vi "IV_Sensor_Check.vi"(10 "Data":dbl[][](array[numeric])=[[1.0, -1.0, 15.0, -15.0], [2.0, -2.0, 30.0, -30.0], [3.0, -3.0, 45.0, -45.0], [4.0, -4.0, 60.0, -60.0]], 11 "Titles":string[](array[string])=["Bias", "Total", "Active", "Guard"]) -> (2 "Boolean Pass/Fail Array":bool[](array[boolean]), 3 "Test Check Names":string[](array[string]))   [LabVIEW 2009]
panel:
  out "Pass/Fail":T1
  out "Passed/Failed Tests":string[](array[string])
  out "Pass":bool
  out "Voltage Breakdown":bool
  out "avg-y 2":dbl
  out "Loop Iteration":i32
  out "avg-y":dbl
  out "avg-x":dbl
  out "Leakage Current Guardring":bool caption="Leakage Current Check Guard"
  out "Leakage Current Check Active":bool
  out "Leakage Current Check Total":bool
  out "150V Bias Check":bool
  out "element 5":dbl
  out "element 4":string
  out "Guadring":dbl[](array[numeric])
  out "element 3":string
  out "Active":dbl[](array[numeric])
  out "element 2":string
  out "Total":dbl[](array[numeric])
  out "element":string
  out "Bias":dbl[](array[numeric])
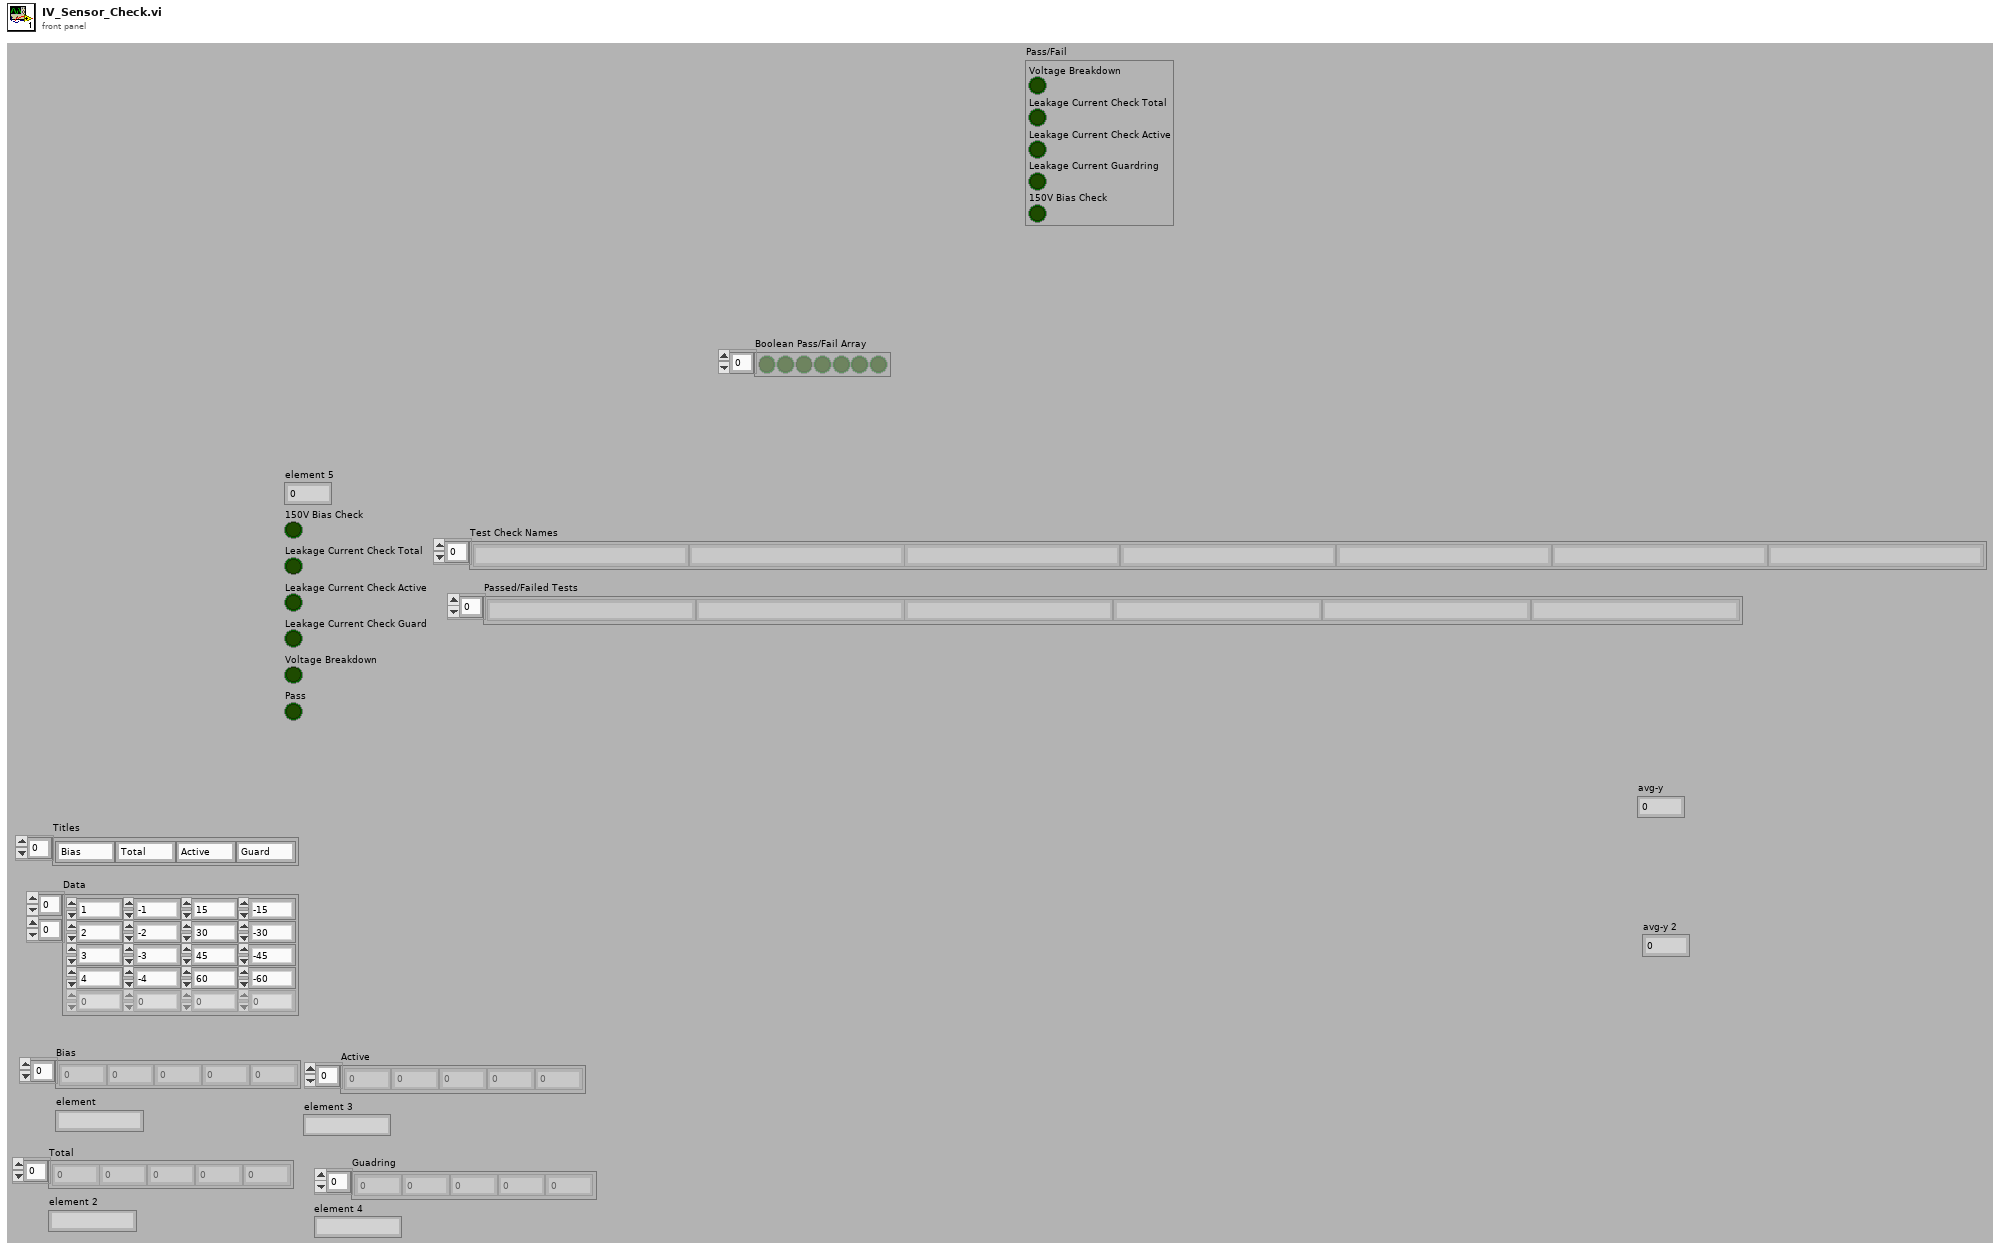
[diagram p1: front panel]
types:
  T1 = cluster{"Voltage Breakdown":bool, "Leakage Current Check Total":bool, "Leakage Current Check Active":bool, "Leakage Current Guardring":bool, "150V Bias Check":bool}
  T2 = cluster{"Numeric":dbl, "Numeric":dbl, "Numeric":dbl, "Numeric":dbl, "Numeric":dbl}
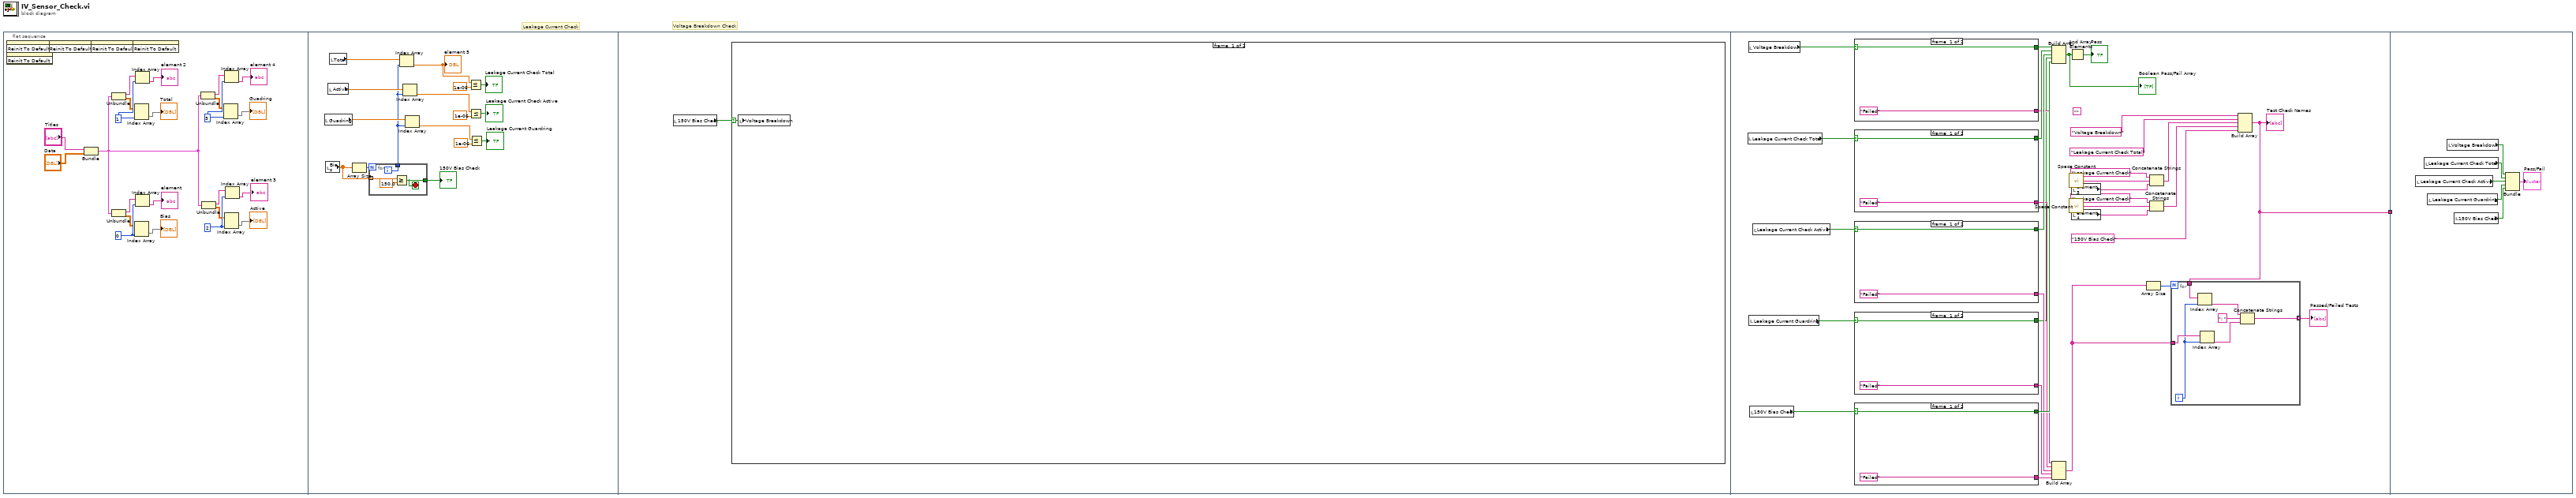
[diagram p0: block diagram]
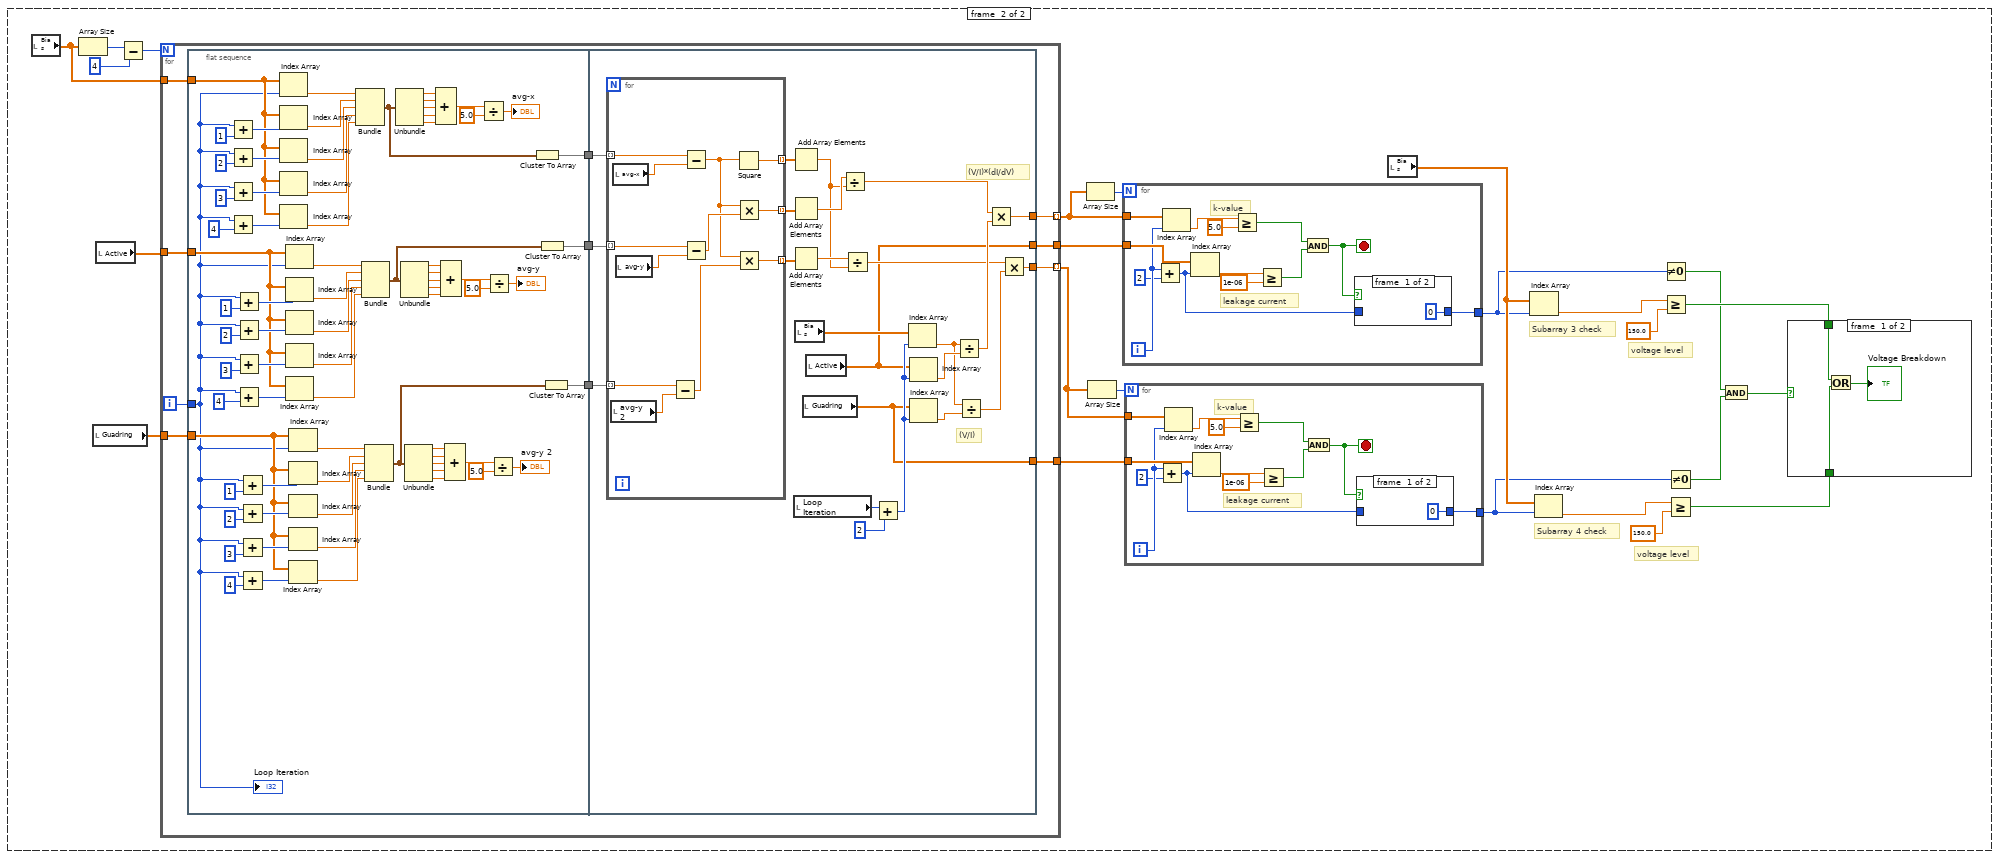
[diagram p2: hidden frame]
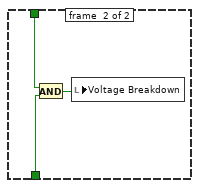
[diagram p3: hidden frame]
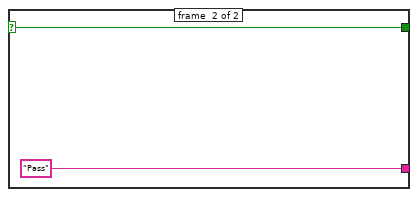
[diagram p6: hidden frame]
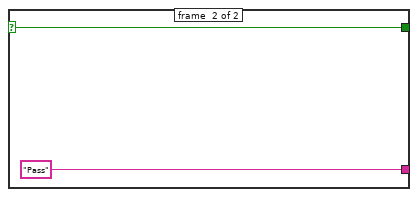
[diagram p7: hidden frame]
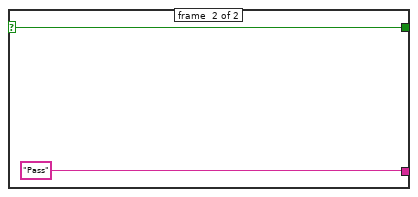
[diagram p8: hidden frame]
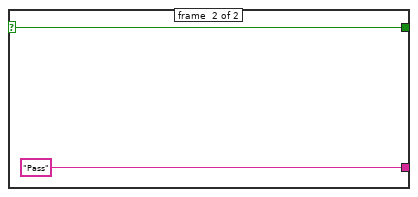
[diagram p9: hidden frame]
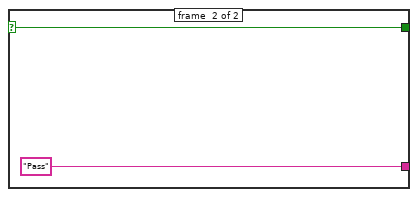
[diagram p10: hidden frame]
diagram:
  # "Voltage Breakdown Check"
  # "Leakage Current Check"
  n1 = flat-sequence {
    tunnel: [w228] -> w1
    tunnel: w1 -> [_]
    frame #0 {
      w23 = u32 3 ("milliseconds to wait")
      w18 = u32 2 ("milliseconds to wait")
      w13 = u32 1 ("milliseconds to wait")
      w8 = u32 0 ("milliseconds to wait")
      n2 = invoke on="Leakage Current Check Total" class="Bool (strict)" method="Reinit To Default"() -> ()  [unwired: 3 in, 3 out]
      n3 = invoke on="Voltage Breakdown" class="Bool (strict)" method="Reinit To Default"() -> ()  [unwired: 3 in, 3 out]
      n4 = invoke on="Leakage Current Check Active" class="Bool (strict)" method="Reinit To Default"() -> ()  [unwired: 3 in, 3 out]
      n5 = Bundle("Titles"="Titles", "Data"="Data") -> (w24:cluster{"Titles":string[], "Data":dbl[][]})  [unwired: 1 in]
      n6 = invoke on="Leakage Current Guardring" class="Bool (strict)" method="Reinit To Default"() -> ()  [unwired: 3 in, 3 out]
      n7 = Unbundle(w24) -> ("Titles"=w11:string[], "Data"=w12:dbl[][])
      n8 = Unbundle(w24) -> ("Titles"=w6:string[], "Data"=w7:dbl[][])
      n9 = invoke on="150V Bias Check" class="Bool (strict)" method="Reinit To Default"() -> ()  [unwired: 3 in, 3 out]
      n10 = Index Array(array=w12, index (col)=w13) -> (element=→"Total":dbl[])  [unwired: 1 in]
      n11 = Index Array(array=w7, index (col)=w8) -> (element=→"Bias":dbl[])  [unwired: 1 in]
      n12 = Index Array(array=w11, index=w13) -> (element=→"element 2":string)
      n13 = Index Array(array=w6, index=w8) -> (element=→"element":string)
      n14 = Unbundle(w24) -> ("Titles"=w21:string[], "Data"=w22:dbl[][])
      n15 = Unbundle(w24) -> ("Titles"=w16:string[], "Data"=w17:dbl[][])
      n16 = Index Array(array=w22, index (col)=w23) -> (element=→"Guadring":dbl[])  [unwired: 1 in]
      n17 = Index Array(array=w17, index (col)=w18) -> (element=→"Active":dbl[])  [unwired: 1 in]
      n18 = Index Array(array=w21, index=w23) -> (element=→"element 4":string)
      n19 = Index Array(array=w16, index=w18) -> (element=→"element 3":string)
    }
    frame #1 {
      n20 = local read "Guadring"() -> (w29:dbl[])
      n21 = local read "Bias"() -> (w39:dbl[])
      n22 = local read "Active"() -> (w33:dbl[])
      n23 = local read "Total"() -> (w34:dbl[])
      n24 = Array Size(array=w39) -> (size(s)=w40:i32)
      n25 = for {
        N: w40 -> [_]
        tunnel: w39 -> [w43] mode=indexing
        tunnel: [w42] -> w28
        tunnel: [w41] -> w38
        i -> [w42]
        stop <- w41 stop-if-true
        n26 = Greater Or Equal?(x=w43, y=150.0 ("element")) -> (x >= y?=w41:bool)
      }
      "150V Bias Check" <- w38
      n27 = Index Array(array=w34, index=w28) -> (element=w37:dbl)
      "element 5" <- w37
      n28 = Index Array(array=w33, index=w28) -> (element=w30:dbl)
      n29 = Index Array(array=w29, index=w28) -> (element=w25:dbl)
      n30 = Less Or Equal?(x=w37, y=1e-06) -> (x <= y?=→"Leakage Current Check Total":bool)
      n31 = Less Or Equal?(x=w30, y=1e-06) -> (x <= y?=→"Leakage Current Check Active":bool)
      n32 = Less Or Equal?(x=w25, y=1e-06) -> (x <= y?=→"Leakage Current Guardring":bool)
    }
    frame #2 {
      n33 = local read "150V Bias Check"() -> (w45:bool)
      n34 = case shown="True" w45 {
        selector: w45 -> [w46 _]
        frame #0 {
          n35 = local write "Voltage Breakdown"(w46) -> ()
        }
        frame #1 {
          # "voltage level"
          # "voltage level"
          # "Subarray 4 check"
          # "Subarray 3 check"
          n36 = local read "Bias"() -> (w67:dbl[])
          n37 = Array Size(array=w67) -> (size(s)=w69:i32)
          n38 = local read "Guadring"() -> (w65:dbl[])
          n39 = local read "Active"() -> (w66:dbl[])
          n40 = Subtract(x=w69, y=4) -> (x-y=w70:i32)
          n41 = for {
            N: w70 -> [_]
            tunnel: w67 -> [w117]
            tunnel: w66 -> [w116]
            tunnel: w65 -> [w112]
            tunnel: [w110] -> w62 mode=indexing
            tunnel: [w109] -> w58 mode=indexing
            tunnel: [w108] -> w64
            tunnel: [w107] -> w60
            i -> [w113]
            n42 = flat-sequence {
              tunnel: w113 -> [w122]
              tunnel: w117 -> [w180]
              tunnel: w116 -> [w150]
              tunnel: [w148] -> w115
              tunnel: [w146] -> w114
              tunnel: w112 -> [w124]
              tunnel: [w123] -> w111
              tunnel: w115 -> [w214]
              tunnel: w114 -> [w213]
              tunnel: w111 -> [w203]
              tunnel: [w194] -> w110
              tunnel: [w193] -> w109
              tunnel: [w192] -> w108
              tunnel: [w191] -> w107
              frame #0 {
                n43 = Add(x=w122, y=1) -> (x+y=w188:i32)
                n44 = Add(x=w122, y=2) -> (x+y=w189:i32)
                n45 = Add(x=w122, y=3) -> (x+y=w190:i32)
                n46 = Add(x=w122, y=4) -> (x+y=w119:i32)
                n47 = Add(x=w122, y=1) -> (x+y=w167:i32)
                n48 = Add(x=w122, y=2) -> (x+y=w168:i32)
                n49 = Add(x=w122, y=3) -> (x+y=w169:i32)
                n50 = Add(x=w122, y=4) -> (x+y=w120:i32)
                n51 = Add(x=w122, y=1) -> (x+y=w143:i32)
                n52 = Add(x=w122, y=2) -> (x+y=w144:i32)
                n53 = Add(x=w122, y=3) -> (x+y=w145:i32)
                n54 = Add(x=w122, y=4) -> (x+y=w121:i32)
                n55 = Index Array(array=w180, index=w122) -> (element=w183:dbl)
                n56 = Index Array(array=w180, index=w188) -> (element=w178:dbl)
                n57 = Index Array(array=w180, index=w189) -> (element=w179:dbl)
                n58 = Index Array(array=w180, index=w190) -> (element=w181:dbl)
                n59 = Index Array(array=w180, index=w119) -> (element=w182:dbl)
                n60 = Index Array(array=w150, index=w122) -> (element=w163:dbl)
                n61 = Index Array(array=w150, index=w167) -> (element=w159:dbl)
                n62 = Index Array(array=w150, index=w168) -> (element=w160:dbl)
                n63 = Index Array(array=w150, index=w169) -> (element=w161:dbl)
                n64 = Index Array(array=w150, index=w120) -> (element=w162:dbl)
                n65 = Index Array(array=w124, index=w122) -> (element=w138:dbl)
                n66 = Index Array(array=w124, index=w143) -> (element=w134:dbl)
                n67 = Index Array(array=w124, index=w144) -> (element=w135:dbl)
                n68 = Index Array(array=w124, index=w145) -> (element=w136:dbl)
                n69 = Index Array(array=w124, index=w121) -> (element=w137:dbl)
                n70 = Bundle("Numeric"=w183, "Numeric"=w178, "Numeric"=w179, "Numeric"=w181, "Numeric"=w182) -> (w149:T2)  [unwired: 1 in]
                n71 = Bundle("Numeric"=w163, "Numeric"=w159, "Numeric"=w160, "Numeric"=w161, "Numeric"=w162) -> (w147:T2)  [unwired: 1 in]
                n72 = Bundle("Numeric"=w138, "Numeric"=w134, "Numeric"=w135, "Numeric"=w136, "Numeric"=w137) -> (w125:T2)  [unwired: 1 in]
                n73 = Unbundle(w149) -> ("Numeric"=w171:dbl, "Numeric"=w172:dbl, "Numeric"=w173:dbl, "Numeric"=w174:dbl, "Numeric"=w175:dbl)
                n74 = Unbundle(w147) -> ("Numeric"=w152:dbl, "Numeric"=w153:dbl, "Numeric"=w154:dbl, "Numeric"=w155:dbl, "Numeric"=w156:dbl)
                n75 = Unbundle(w125) -> ("Numeric"=w127:dbl, "Numeric"=w128:dbl, "Numeric"=w129:dbl, "Numeric"=w130:dbl, "Numeric"=w131:dbl)
                n76 = Compound Arithmetic op=ADD(w171, w172, w173, w174, w175) -> (w170:dbl)
                n77 = Compound Arithmetic op=ADD(w152, w153, w154, w155, w156) -> (w151:dbl)
                n78 = Compound Arithmetic op=ADD(w127, w128, w129, w130, w131) -> (w126:dbl)
                n79 = Divide(x=w170, y=5.0) -> (x/y=→"avg-x":dbl)
                n80 = Divide(x=w151, y=5.0) -> (x/y=→"avg-y":dbl)
                n81 = Divide(x=w126, y=5.0) -> (x/y=→"avg-y 2":dbl)
                n82 = Cluster To Array(cluster=w149) -> (array=w148:dbl[])
                n83 = Cluster To Array(cluster=w147) -> (array=w146:dbl[])
                n84 = Cluster To Array(cluster=w125) -> (array=w123:dbl[])
                "Loop Iteration" <- w122
              }
              frame #1 {
                # "(V/I)*(dI/dV)"
                # "(V/I)"
                n85 = for {
                  tunnel: w214 -> [w226] mode=indexing
                  tunnel: w213 -> [w224] mode=indexing
                  tunnel: [w221] -> w212 mode=indexing
                  tunnel: [w220] -> w211 mode=indexing
                  tunnel: w203 -> [w219] mode=indexing
                  tunnel: [w215] -> w201 mode=indexing
                  n86 = local read "avg-y 2"() -> (w218:dbl)
                  n87 = local read "avg-x"() -> (w225:dbl)
                  n88 = local read "avg-y"() -> (w223:dbl)
                  n89 = Subtract(x=w219, y=w218) -> (x-y=w216:dbl)
                  n90 = Subtract(x=w226, y=w225) -> (x-y=w217:dbl)
                  n91 = Subtract(x=w224, y=w223) -> (x-y=w222:dbl)
                  n92 = Square(x=w217) -> (x^2=w221:dbl)
                  n93 = Multiply(x=w217, y=w222) -> (x*y=w220:dbl)
                  n94 = Multiply(x=w217, y=w216) -> (x*y=w215:dbl)
                }
                n95 = Add Array Elements(numeric array=w212) -> (sum=w199:dbl)
                n96 = Add Array Elements(numeric array=w211) -> (sum=w210:dbl)
                n97 = Add Array Elements(numeric array=w201) -> (sum=w200:dbl)
                n98 = local read "Loop Iteration"() -> (w209:i32)
                n99 = local read "Bias"() -> (w207:dbl[])
                n100 = local read "Guadring"() -> (w191:dbl[])
                n101 = local read "Active"() -> (w192:dbl[])
                n102 = Divide(x=w210, y=w199) -> (x/y=w205:dbl)
                n103 = Divide(x=w200, y=w199) -> (x/y=w196:dbl)
                n104 = Add(x=w209, y=2) -> (x+y=w202:i32)
                n105 = Index Array(array=w207, index=w202) -> (element=w197:dbl)
                n106 = Index Array(array=w192, index=w202) -> (element=w206:dbl)
                n107 = Index Array(array=w191, index=w202) -> (element=w198:dbl)
                n108 = Divide(x=w197, y=w206) -> (x/y=w204:dbl)
                n109 = Divide(x=w197, y=w198) -> (x/y=w195:dbl)
                n110 = Multiply(x=w205, y=w204) -> (x*y=w194:dbl)
                n111 = Multiply(x=w196, y=w195) -> (x*y=w193:dbl)
              }
            }
          }
          n112 = Array Size(array=w62) -> (size(s)=w63:i32)
          n113 = Array Size(array=w58) -> (size(s)=w59:i32)
          n114 = for {
            N: w63 -> [_]
            tunnel: w62 -> [w104]
            tunnel: w64 -> [w103]
            tunnel: [w93] -> w52
            i -> [w102]
            stop <- w92 stop-if-true
            # "leakage current"
            # "k-value"
            n115 = Add(x=w102, y=2) -> (x+y=w94:i32)
            n116 = Index Array(array=w104, index=w102) -> (element=w100:dbl)
            n117 = Index Array(array=w103, index=w94) -> (element=w99:dbl)
            n118 = Greater Or Equal?(x=w100, y=5.0) -> (x >= y?=w98:bool)
            n119 = Greater Or Equal?(x=w99, y=1e-06) -> (x >= y?=w97:bool)
            n120 = And(x=w98, y=w97) -> (x .and. y?=w92:bool)
            n121 = case shown="False" w92 {
              tunnel: w94 -> [_ w106]
              tunnel: [0 w106] -> w93
              frame #0 {
              }
              frame #1 {
              }
            }
          }
          n122 = for {
            N: w59 -> [_]
            tunnel: w58 -> [w89]
            tunnel: w60 -> [w88]
            tunnel: [w78] -> w53
            i -> [w87]
            stop <- w77 stop-if-true
            # "leakage current"
            # "k-value"
            n123 = Add(x=w87, y=2) -> (x+y=w79:i32)
            n124 = Index Array(array=w89, index=w87) -> (element=w85:dbl)
            n125 = Index Array(array=w88, index=w79) -> (element=w84:dbl)
            n126 = Greater Or Equal?(x=w85, y=5.0) -> (x >= y?=w83:bool)
            n127 = Greater Or Equal?(x=w84, y=1e-06) -> (x >= y?=w82:bool)
            n128 = And(x=w83, y=w82) -> (x .and. y?=w77:bool)
            n129 = case shown="False" w77 {
              tunnel: w79 -> [_ w91]
              tunnel: [0 w91] -> w78
              frame #0 {
              }
              frame #1 {
              }
            }
          }
          n130 = local read "Bias"() -> (w56:dbl[])
          n131 = Index Array(array=w56, index=w52) -> (element=w55:dbl)
          n132 = Index Array(array=w56, index=w53) -> (element=w54:dbl)
          n133 = Not Equal To 0?(x=w52) -> (x != 0?=w49:bool)
          n134 = Greater Or Equal?(x=w55, y=150.0) -> (x >= y?=w51:bool)
          n135 = Not Equal To 0?(x=w53) -> (x != 0?=w48:bool)
          n136 = Greater Or Equal?(x=w54, y=150.0) -> (x >= y?=w50:bool)
          n137 = And(x=w49, y=w48) -> (x .and. y?=w47:bool)
          n138 = case shown="False" w47 {
            tunnel: w51 -> [w72 w75]
            tunnel: w50 -> [w71 w74]
            frame #0 {
              n139 = Or(x=w72, y=w71) -> (x .or. y?=→"Voltage Breakdown":bool)
            }
            frame #1 {
              n140 = And(x=w75, y=w74) -> (x .and. y?=w76:bool)
              n141 = local write "Voltage Breakdown"(w76) -> ()
            }
          }
        }
      }
    }
    frame #3 {
      (unwired) ""
      n142 = local read "Leakage Current Check Total"() -> (w257:bool)
      n143 = local read "Voltage Breakdown"() -> (w258:bool)
      n144 = local read "Leakage Current Guardring"() -> (w255:bool)
      n145 = local read "150V Bias Check"() -> (w256:bool)
      n146 = local read "Leakage Current Check Active"() -> (w254:bool)
      n147 = case shown="False" w258 {
        selector: w258 -> [w283 w285]
        tunnel: [w283 w285] -> w253
        tunnel: ["Failed" "Pass"] -> w244
        frame #0 {
        }
        frame #1 {
        }
      }
      n148 = case shown="False" w257 {
        selector: w257 -> [w279 w281]
        tunnel: [w279 w281] -> w252
        tunnel: ["Failed" "Pass"] -> w245
        frame #0 {
        }
        frame #1 {
        }
      }
      n149 = case shown="False" w254 {
        selector: w254 -> [w267 w269]
        tunnel: [w267 w269] -> w251
        tunnel: ["Failed" "Pass"] -> w246
        frame #0 {
        }
        frame #1 {
        }
      }
      n150 = case shown="False" w255 {
        selector: w255 -> [w271 w273]
        tunnel: [w271 w273] -> w227
        tunnel: ["Failed" "Pass"] -> w247
        frame #0 {
        }
        frame #1 {
        }
      }
      n151 = case shown="False" w256 {
        selector: w256 -> [w275 w277]
        tunnel: [w275 w277] -> w250
        tunnel: ["Failed" "Pass"] -> w248
        frame #0 {
        }
        frame #1 {
        }
      }
      n152 = Build Array(w253, w252, w251, w227, w250) -> (w229:bool[])
      "Boolean Pass/Fail Array" <- w229
      n153 = Build Array(w244, w245, w246, w247, w248) -> (w231:string[])
      n154 = call <vilib>:"Space Constant.vi"() -> ("String"=w242:string)
      n155 = call <vilib>:"Space Constant.vi"() -> ("String"=w239:string)
      n156 = And Array Elements(Boolean array=w229) -> (logical AND=→"Pass":bool)
      n157 = local read "element 3"() -> (w241:string)
      n158 = local read "element 4"() -> (w238:string)
      n159 = Array Size(array=w231) -> (size(s)=w232:i32)
      n160 = Concatenate Strings("Leakage Current Check", w242, w241) -> (w235:string)
      n161 = Concatenate Strings("Leakage Current Check", w239, w238) -> (w234:string)
      n162 = Build Array("Voltage Breakdown", "Leakage Current Check Total", w235, w234, "150V Bias Check") -> (w228:string[])
      "Test Check Names" <- w228
      n163 = for {
        N: w232 -> [_]
        tunnel: w228 -> [w265]
        tunnel: w231 -> [w264]
        tunnel: [w260] -> w230 mode=indexing
        i -> [w259]
        n164 = Index Array(array=w265, index=w259) -> (element=w263:string)
        n165 = Index Array(array=w264, index=w259) -> (element=w262:string)
        n166 = Concatenate Strings(w263, ": " ("string"), w262) -> (w260:string)
      }
      "Passed/Failed Tests" <- w230
    }
    frame #4 {
      n167 = local read "Leakage Current Check Active"() -> (w289:bool)
      n168 = local read "Leakage Current Check Total"() -> (w290:bool)
      n169 = local read "Leakage Current Guardring"() -> (w288:bool)
      n170 = local read "Voltage Breakdown"() -> (w291:bool)
      n171 = local read "150V Bias Check"() -> (w287:bool)
      n172 = Bundle("Voltage Breakdown"=w291, "Leakage Current Check Total"=w290, "Leakage Current Check Active"=w289, "Leakage Current Guardring"=w288, "150V Bias Check"=w287) -> (→"Pass/Fail":T1)  [unwired: 1 in]
    }
  }
